vi "Create Section Group.vi"(8 "error in":errorcluster, 11 "Group Scalar Data in":T1 {"Scalar Section ref" format="%.0x"; "Group Section ref" format="%.0x"; "Group Scalar Registers"."Data Type" format="%.0x"}) -> (0 "error out":errorcluster, 3 "Group Scalar Data out":T1 {"Scalar Section ref" format="%.0x"; "Group Section ref" format="%.0x"; "Group Scalar Registers"."Data Type" format="%.0x"})   [LabVIEW 2020, in "Scripting API.lvlib"]
uses:
  Scripting API.lvlib
  TypeDefs/Group Scalar Data.ctl
  <vilib>/NI VeriStand/Custom Device API/Custom Device Item Ref.ctl
  Addon/Addon Shared/Types/Register Information.ctl
  Addon/Addon Shared/Types/FPGA Addon Data Type.ctl
  Addon/Addon Shared/Types/FG Action.ctl
  Addon/Addon Shared/SubVIs/Constants.vi
  <vilib>/NI/NI VeriStand Advanced SysDef API/SysDef API/SysDef.Property.Get.vi
  <vilib>/NI/NI VeriStand Advanced SysDef API/_SubVIs/SysDef.Property.Get.Variant.vi
  <vilib>/NI/NI VeriStand Advanced SysDef API/SysDef API/SysDef.Property.Set.vi
  <vilib>/NI/NI VeriStand Advanced SysDef API/_SubVIs/SysDef.Property.Set.Variant.vi
  <vilib>/NI VeriStand/Custom Device API/Custom Device API.lvlib
  Addon/Addon Shared/FPGA Addon Shared.lvlib
  Addon/Addon System Explorer/FPGA Addon System Explorer.lvlib
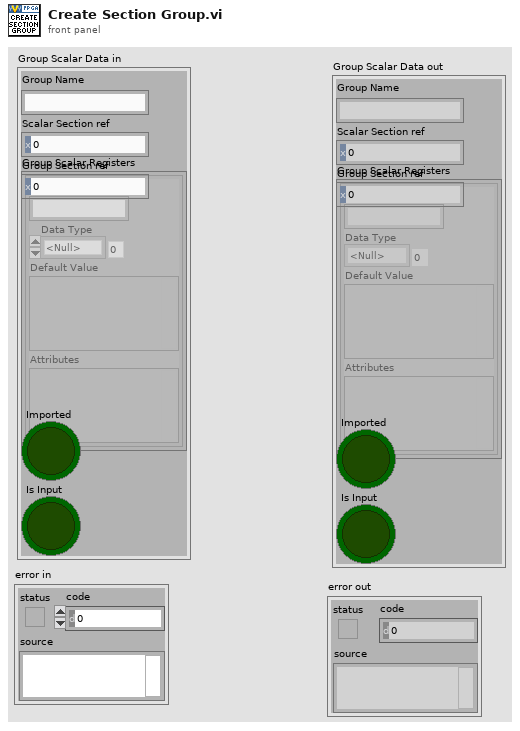
[diagram p1: front panel]
types:
  T1 = typedef "Scripting API.lvlib/Group Scalar Data.ctl" = cluster{"Group Name":string, "Scalar Section ref":T2, "Group Section ref":T2, "Group Scalar Registers":T3[], "Imported":bool, "Is Input":bool}
  T2 = typedef "Custom Device API.lvlib/Custom Device Item Ref.ctl" = u64
  T3 = typedef "FPGA Addon Shared.lvlib/Register Information.ctl" = cluster{"Name":string, "Data Type":T4, "Default Value":variant, "Attributes":variant}
  T4 = typedef "FPGA Addon Shared.lvlib/FPGA Addon Data Type.ctl" = enum8{"<Null>", "I8", "I16", "I32", "I64", "U8", "U16", "U32", "U64", "SGL", "Boolean", "Analog PWM In Settings", "Analog PWM In", "Digital PWM In Settings", "Digital PWM In", "Digital PWM Out", "Sine Out", "FXP", "FXP+/-24.5", "FXP+/-16.5", "FXP+/-32.8", "FXP+/-64.32", "FXP+/-16.7", "FXP+/-20.5", "FXP+/-27.5", "FXP+/-32.16", "FXP+16.3", "FXP+18.3", "Digital Static In", "Digital Static Out", "Digital Static In Settings", "Digital WSS Out", "Quad Encoder Settings", "Quad Encoder In", "Group"}
  T5 = typedef "FPGA Addon Shared.lvlib/FG Action.ctl" = enum8{"GET", "SET"}
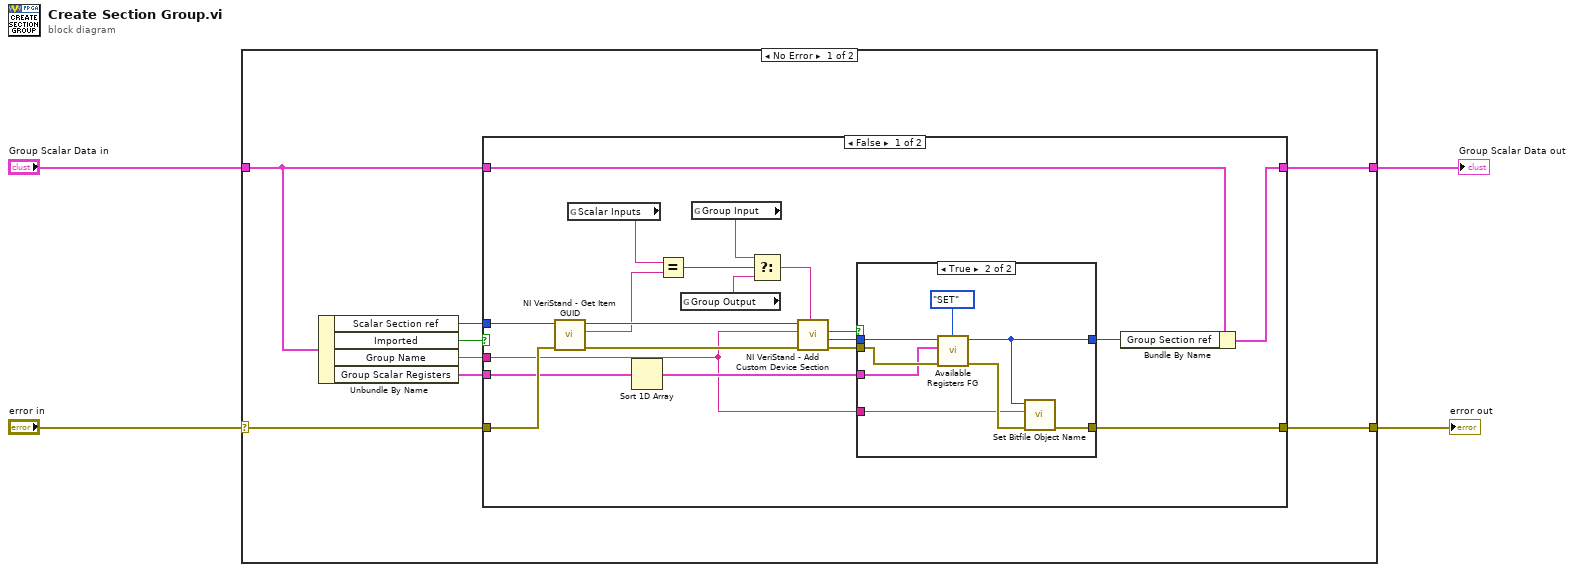
[diagram p0: block diagram]
diagram:
  n1 = case shown="No Error" "error in" {
    selector: "error in" -> [w8 w46]
    tunnel: "Group Scalar Data in" -> [w12 w45]
    tunnel: [w9 w45] -> w3
    tunnel: [w7 w46] -> w1
    frame No Error {
      n2 = Unbundle By Name(w12) -> ("Scalar Section ref"=w11:T2, "Imported"=w10:bool, "Group Name"=w5:string, "Group Scalar Registers"=w6:T3[])
      n3 = case shown="False" w10 {
        tunnel: w11 -> [w30 _]
        tunnel: w12 -> [w32 w44]
        tunnel: [w31 w44] -> w9
        tunnel: w8 -> [w25 w43]
        tunnel: [w19 w43] -> w7
        tunnel: w6 -> [w15 _]
        tunnel: w5 -> [w13 _]
        frame False {
          n4 = call <vilib>:"NI VeriStand - Get Item GUID.vi"("error in (no error)"=w25, "Item Ref in"=w30) -> ("error out"=w24:errorcluster, "GUID"=w18:string, "Item Ref out"=w26:T2)  [unwired: 7 in]
          n5 = global read "Constants.vi" "Scalar Inputs"() -> (w17:string)
          n6 = Sort 1D Array(array=w15) -> (sorted array=w14:T3[])
          n7 = Equal?(x=w17, y=w18) -> (x = y?=w29:bool)
          n8 = global read "Constants.vi" "Group Output"() -> (w27:string)
          n9 = global read "Constants.vi" "Group Input"() -> (w28:string)
          n10 = Select(t=w28, s=w29, f=w27) -> (s? t:f=w23:string)
          n11 = call <vilib>:"NI VeriStand - Add Custom Device Section.vi"("GUID (Default Section)"=w23, "error in (no error)"=w24, "Section Name"=w13, "Parent Ref in"=w26) -> ("error out"=w21:errorcluster, "Section Ptr"=w22:T2, "Newly Created?"=w16:bool)  [unwired: 4 in, 1 out]
          n12 = case shown="True" w16 {
            tunnel: w22 -> [w34 w41]
            tunnel: w21 -> [w33 w40]
            tunnel: [w34 w37] -> w20
            tunnel: [w33 w36] -> w19
            tunnel: w14 -> [_ w39]
            tunnel: w13 -> [_ w35]
            frame False {
            }
            frame True {
              n13 = call "Available Registers FG.vi"("Action"=FG_Action."SET", "error in (no error)"=w40, "Available Registers"=w39, "Item Ref"=w41) -> ("error out"=w38:errorcluster, "Item Ref out"=w37:T2)  [unwired: 5 in, 1 out]
              n14 = call "Set Bitfile Object Name.vi"("error in (no error)"=w38, "Name"=w35, "Channel Ref"=w37) -> ("error out"=w36:errorcluster)  [unwired: 8 in]
            }
          }
          n15 = Bundle By Name(cluster=w32, "Group Section ref"=w20) -> (w31:T1)
        }
        frame True {
        }
      }
    }
    frame Error {
    }
  }
  "Group Scalar Data out" <- w3
  "error out" <- w1
